vi "Write discover channels.vi"(8 "error in":errorcluster, 10 "discover channels":bool, 11 "Scan Engine configuration in":refnum<class "Scan Engine configuration.lvclass">) -> (0 "error out":errorcluster, 3 "Scan Engine configuration out":refnum<class "Scan Engine configuration.lvclass">)   [LabVIEW 2013, in "Scan Engine configuration.lvclass"]
uses:
  Scan Engine configuration.lvclass
  Scan Engine configuration.lvclass/Scan Engine configuration.ctl
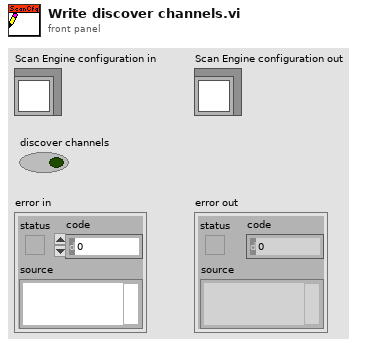
[diagram p1: front panel]
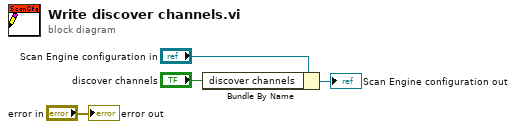
[diagram p0: block diagram]
diagram:
  n1 = Bundle By Name(cluster="Scan Engine configuration in", "discover channels"="discover channels") -> (→"Scan Engine configuration out":refnum<class "Scan Engine configuration.lvclass">)
  "error out" <- "error in"
